vi "Update_UI_Overlay.vi"(8 "error in (no error)":errorcluster, 11 "Image Refnum":refnum<vi>) -> (0 "error out":errorcluster)   [LabVIEW 2019]
uses:
  Controls/ROI_List_Action.ctl
  <vilib>/vision/Image Controls.llb/IMAQ Image.ctl
panel:
  in  "Vision_Image":T1(plugin-control)
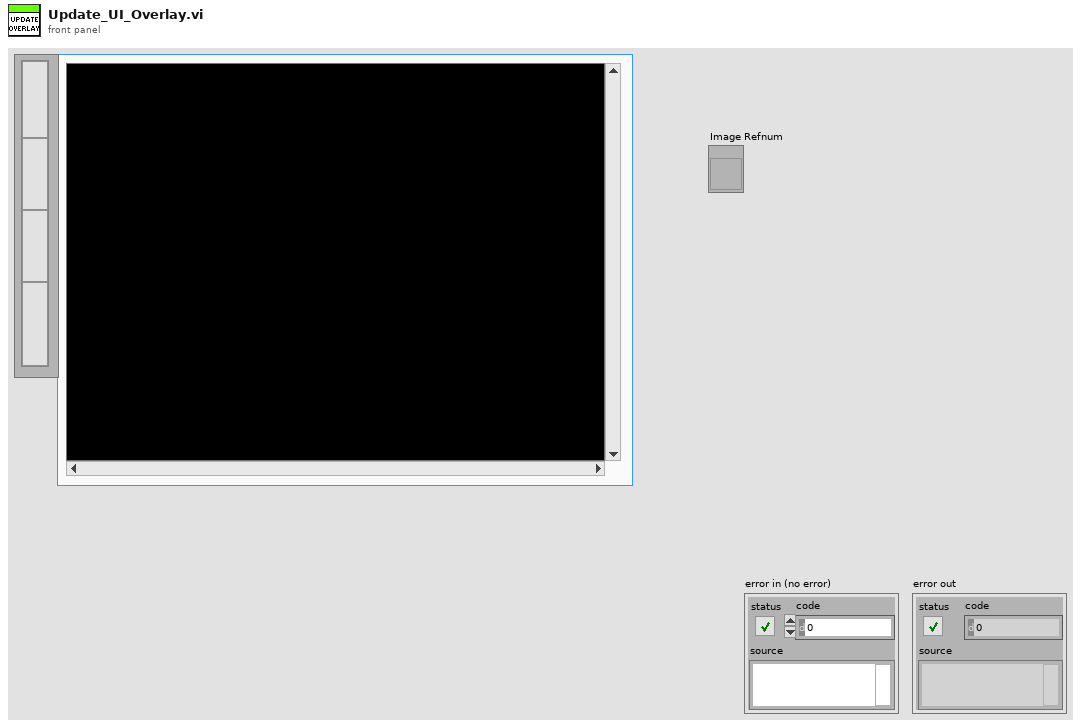
[diagram p1: front panel]
types:
  T1 = typedef "IMAQ Image.ctl" = refnum<image>
  T2 = typedef "ROI_List_Action.ctl" = enum16{"Init", "Add ROI", "Delete ROI", "Get All ROI", "Get Specific ROI", "Set Analysis Setting", "Set Process Setting", "Replace All Entries", "ROIEntryBackup", "ROIEntryBackupClear", "ROIEntryReturn"}
  T3 = typedef "Vision_DataEntry.ctl" = cluster{"vROIName":string, "vROIContour":cluster{"Contour Type":u32, "ROI Type":u32, "Points":i32[]}, "ProcessSetting":T4[], "Analysis_Setting":T6}
  T4 = typedef "Process_Setting.ctl" = cluster{"Enum_PreProcess":T5, "Parameter":string}
  T5 = typedef "VisionProcessName.ctl" = enum16{"*CamParameter*", "CamAttributes", "*Preprocess*", "CG_Brightness", "C_Plane Extraction", "C_Threshold", "G_Lookup Table", "G_Threshold"}
  T6 = typedef "Analysis_Setting.ctl" = cluster{"PreProcess":T7, "Parameter":string}
  T7 = typedef "V_Analysis_Type.ctl" = enum16{"None", "C_Color Pattern Matching", "G_PatternMatching", "G_ShapeDectect", "G_GeometricMatch", "B_Area Check"}
  T8 = cluster{"Points[0]":i32, "Points[1]":i32, "Points[2]":i32, "Points[3]":i32}
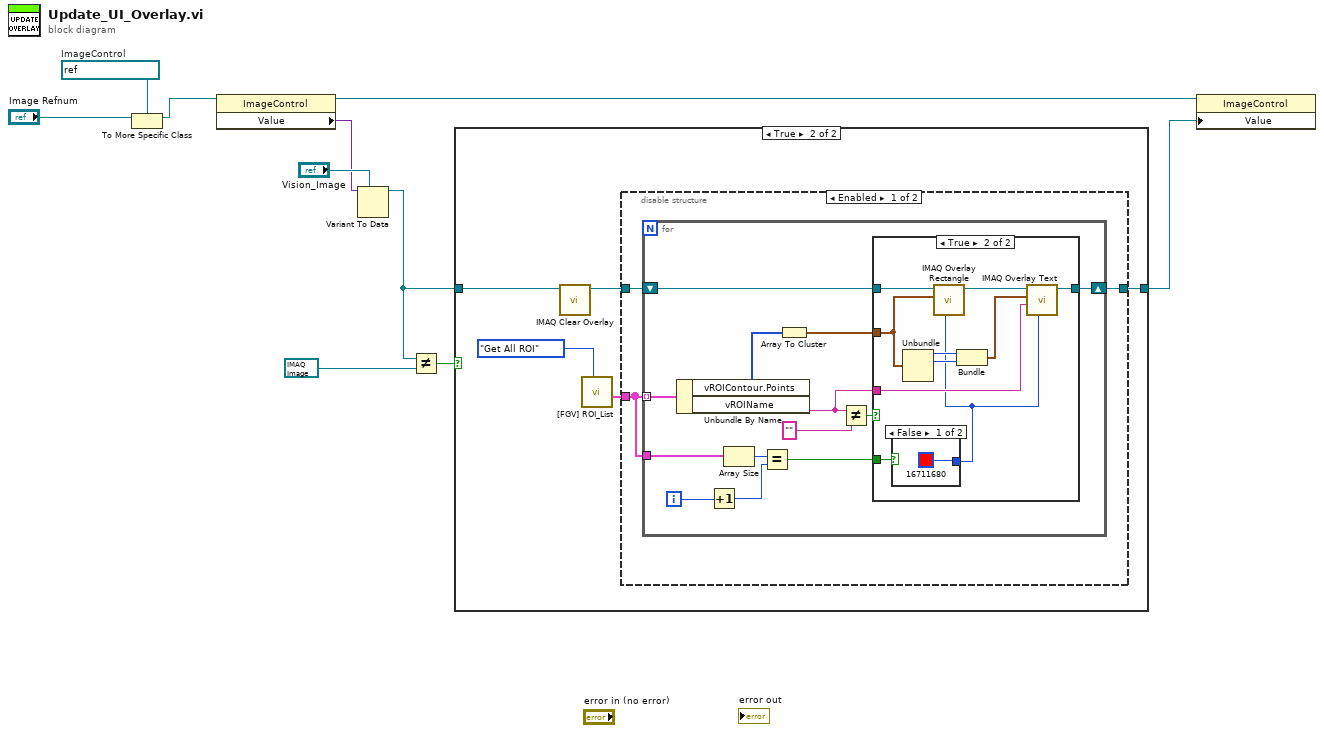
[diagram p0: block diagram]
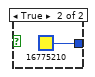
[diagram p4: hidden frame]
diagram:
  w9 = refnum<vi> refnum  # ImageControl
  n1 = To More Specific Class(target class=w9, reference="Image Refnum") -> (specific class reference=w8:refnum<vi>)  [unwired: 1 in, 1 out]
  n2 = property class="ImageControl"(reference=w8) -> (reference out=w7:refnum<vi>, "Value"=w4:variant)  [unwired: 1 in, 1 out]
  n3 = Variant To Data(type="Vision_Image", Variant=w4) -> (data=w3:T1)  [unwired: 1 in, 1 out]
  n4 = Not Equal?(x=w3, y=T1 refnum ("Image Out")) -> (x != y?=w1:bool)
  n5 = case shown="True" w1 {
    tunnel: [w11 w14] -> w6
    tunnel: w3 -> [w11 w13]
    frame False {
    }
    frame True {
      n6 = call "IMAQ Clear Overlay"("Image"=w13) -> ("Image Out"=w12:T1)  [unwired: 9 in, 1 out]
      n7 = call "[FGV] ROI_List.vi"("Action"=ROI_List_Action."Get All ROI") -> ("All ROI"=w15:T3[])  [unwired: 8 in, 2 out]
      n8 = disable-structure shown="Enabled" {
        disable-tunnel: w15 -> [w17 _]
        disable-tunnel: w12 -> [w19 _]
        disable-tunnel: [w18 _] -> w14
        frame Enabled {
          n9 = for {
            tunnel: w17 -> [w30] mode=indexing
            shift-right: [w31] -> w18
            shift-left: w19 -> [w32]
            tunnel: w17 -> [w24]
            i -> [w23]
            n10 = Unbundle By Name(w30) -> ("vROIContour.Points"=w27:i32[], "vROIName"=w25:string)
            n11 = Increment(x=w23) -> (x+1=w21:i32)
            n12 = Array Size(array=w24) -> (size(s)=w22:i32)
            n13 = Equal?(x=w22, y=w21) -> (x = y?=w20:bool)
            n14 = Array To Cluster(array=w27) -> (cluster=w26:T8)
            n15 = Not Equal?(x=w25, y="") -> (x != y?=w28:bool)
            n16 = case shown="True" w28 {
              tunnel: w32 -> [w33 w43]
              tunnel: [w33 w41] -> w31
              tunnel: w26 -> [_ w39]
              tunnel: w25 -> [_ w40]
              tunnel: w20 -> [_ w35]
              frame False {
              }
              frame True {
                n17 = case shown="False" w35 {
                  tunnel: [u32 16711680 ("Text Color (black)") u32 16775210 ("Text Color (black)")] -> w34
                  frame False {
                  }
                  frame True {
                  }
                }
                n18 = Unbundle(w39) -> ("Points[0]"=w38:i32, "Points[1]"=w37:i32)  [unwired: 2 out]
                n19 = call "IMAQ Overlay Rectangle"("Color"=w34, "Rectangle"=w39, "Image"=w43) -> ("Image Out"=w42:T1)  [unwired: 7 in, 1 out]
                n20 = Bundle("Points[0]"=w38, "Points[1]"=w37) -> (w36:cluster{"Points[0]":i32, "Points[1]":i32})  [unwired: 1 in]
                n21 = call "IMAQ Overlay Text"("Text Color (black)"=w34, "String"=w40, "Origin"=w36, "Image"=w42) -> ("Image Out"=w41:T1)  [unwired: 6 in, 1 out]
              }
            }
          }
        }
        frame Disabled {
        }
      }
    }
  }
  n22 = property class="ImageControl"(reference=w7, "Value"=w6) -> ()  [unwired: 1 in, 2 out]
